vi "Check SSH Connection Status.vi"(8 "Error In":errorcluster, 11 "Install LV Data in":T1={"SSH Session"=refnum, "Status Log"="", "Detailed Log"="", "Credentials"={"Hostname or IP"="192.168.7.2", "Username"="root", "Password"=""}, "Target Info"={"OS Version"="", "CPU"="", "Systemd Version"="", "Internet Access"=FALSE, "Device Type"="", "LV Installed Ver"="", "LV Available Ver"="", "LV Upgrade Available"=FALSE, "Hostname"="", "NIC Info"=[]}, "Reboot Required?"=FALSE}) -> (0 "Error Out":errorcluster, 2 "IsConnected":bool, 3 "Install LV Data":T1={"SSH Session"=refnum, "Status Log"="", "Detailed Log"="", "Credentials"={"Hostname or IP"="192.168.7.2", "Username"="root", "Password"=""}, "Target Info"={"OS Version"="", "CPU"="", "Systemd Version"="", "Internet Access"=FALSE, "Device Type"="", "LV Installed Ver"="", "LV Available Ver"="", "LV Upgrade Available"=FALSE, "Hostname"="", "NIC Info"=[]}, "Reboot Required?"=FALSE})   [LabVIEW 2020, in "LMH-LINX.lvlib"]
uses:
  LMH-LINX.lvlib
  Install LV Data.ctl
  Target Info.ctl
  NIC Info.ctl
  NIC Mode.ctl
  c:/p4/penguin/lvaddon/MakerHub/LINX/trunk/20.1/objects/MakerHub_LINX/win32U/i386/msvc90/release/LabVIEW/vi.lib/MakerHub/LINX/Resources/Renci.SshNet.dll
  Resources/Renci.SshNet.dll
  <vilib>/MakerHub/LINX/Private/Utilties/SSH/SSH Unix Session Op.ctl
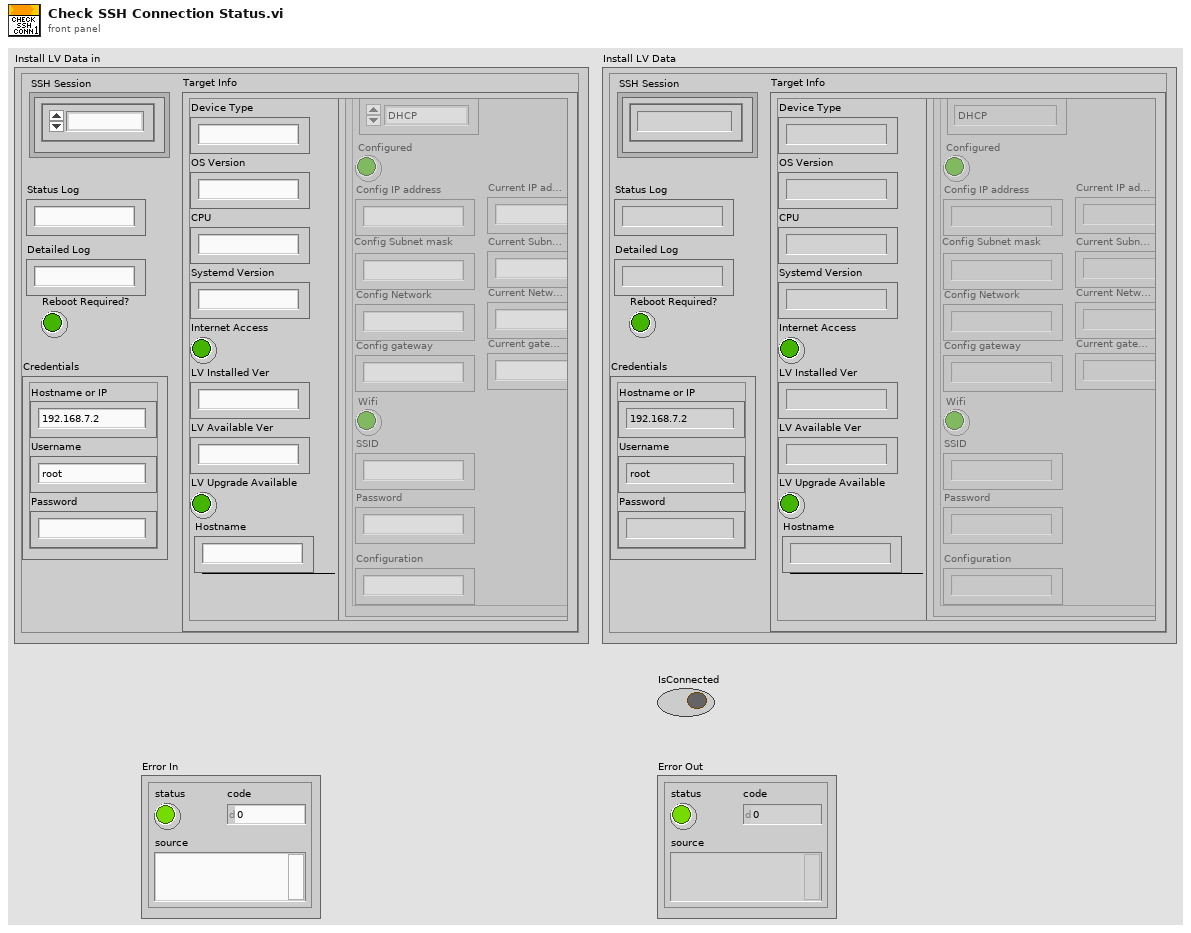
[diagram p1: front panel]
types:
  T1 = typedef "LMH-LINX.lvlib/Install LV Data.ctl" = cluster{"SSH Session":refnum<k1>, "Status Log":string, "Detailed Log":string, "Credentials":cluster{"Hostname or IP":string, "Username":string, "Password":string}, "Target Info":T2, "Reboot Required?":bool}
  T2 = typedef "LMH-LINX.lvlib/Target Info.ctl" = cluster{"OS Version":string, "CPU":string, "Systemd Version":string, "Internet Access":bool, "Device Type":string, "LV Installed Ver":string, "LV Available Ver":string, "LV Upgrade Available":bool, "Hostname":string, "NIC Info":T3[]}
  T3 = typedef "LMH-LINX.lvlib/NIC Info.ctl" = cluster{"Name":string, "NIC Mode":T4, "Configured":bool, "Config IP address":string, "Config Subnet mask":string, "Config Network":string, "Config gateway":string, "Wifi":bool, "SSID":string, "Password":string, "Configuration":string, "Current IP address":string, "Current Subnet mask":string, "Current gateway":string, "Current Network":string}
  T4 = typedef "LMH-LINX.lvlib/NIC Mode.ctl" = enum16{"DHCP", "Static", "Loopback"}
  T5 = typedef "LMH-LINX.lvlib/SSH Unix Session Op.ctl" = enum16{"New", "Get", "Delete"}
  T6 = typedef "LMH-LINX.lvlib/SSH Unix Session Info.ctl" = cluster{"PID":i32, "Read FD":i32, "Write FD":i32, "Error FD":i32}
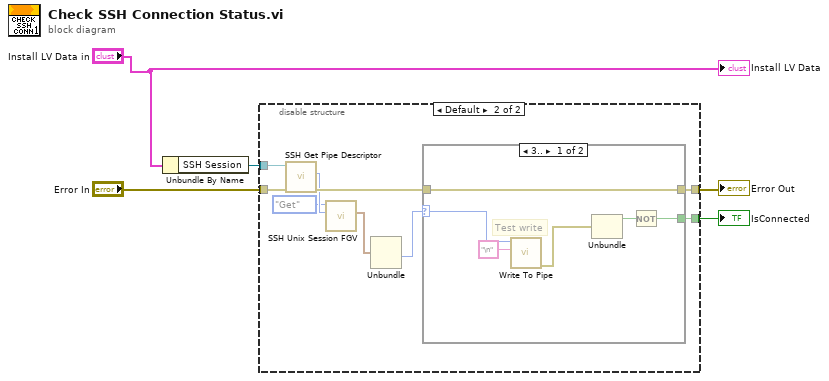
[diagram p0: block diagram]
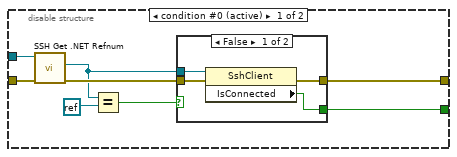
[diagram p2: hidden frame]
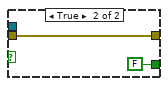
[diagram p3: hidden frame]
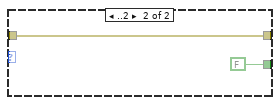
[diagram p4: hidden frame]
diagram:
  n1 = Unbundle By Name("Install LV Data in") -> ("SSH Session"=w1:refnum<k1>)
  n2 = disable-structure shown="Default" {
    disable-tunnel: [w13 w28] -> w5
    disable-tunnel: [w12 w27] -> w4
    disable-tunnel: "Error In" -> [w11 w26]
    disable-tunnel: w1 -> [w10 w25]
    frame condition #0 (active) {
      n3 = call "SSH Get .NET Refnum.vi"("Error In"=w11, "SSH Session"=w10) -> ("Error Out"=w8:errorcluster, "SSH .NET Refnum"=w7:refnum<k24>)  [unwired: 7 in, 1 out]
      n4 = Equal?(x=w7, y=refnum<k0> refnum) -> (x = y?=w6:bool)
      n5 = case shown="False" w6 {
        tunnel: [w17 FALSE ("IsConnected")] -> w13
        tunnel: [w16 w18] -> w12
        tunnel: w8 -> [w15 w18]
        tunnel: w7 -> [w14 _]
        frame False {
          n6 = property class="SshClient"(reference=w14, error in=w15) -> (error out=w16:errorcluster, "IsConnected"=w17:bool)  [unwired: 1 out]
        }
        frame True {
        }
      }
    }
    frame condition #1 {
      n7 = call <vilib>:"SSH Get Pipe Descriptor.vi"("Error In"=w26, "SSH Session"=w25) -> ("Error Out"=w24:errorcluster, "SSH Pipe Descriptor"=w23:i32)  [unwired: 7 in, 1 out]
      n8 = call <vilib>:"SSH Unix Session FGV.vi"("Session In"=w23, "Operation"=SSH_Unix_Session_Op."Get") -> ("info in"=w21:T6)  [unwired: 8 in, 1 out]
      n9 = Unbundle(w21) -> ("Write FD"=w20:i32)  [unwired: 3 out]
      n10 = case shown="3.." w20 {
        selector: w20 -> [w33 _]
        tunnel: [w30 FALSE ("IsConnected")] -> w28
        tunnel: [w29 w35] -> w27
        tunnel: w24 -> [w29 w35]
        frame 3.. {
          # "Test write"
          n11 = call <vilib>:"Write To Pipe.vi"("data"="\n", "file descriptor"=w33) -> ("error out"=w32:errorcluster)  [unwired: 3 in, 2 out]
          n12 = Unbundle(w32) -> ("status"=w31:bool)  [unwired: 2 out]
          n13 = Not(x=w31) -> (.not. x?=w30:bool)
        }
        frame ..2 {
        }
      }
    }
  }
  "IsConnected" <- w5
  "Error Out" <- w4
  "Install LV Data" <- "Install LV Data in"
